vi "MotorInterfaceV2.vi"() -> ()   [LabVIEW 2020]
uses:
  <vilib>/DAQmx/write.llb/DAQmx Write (Digital 1D U16 1Chan NSamp).vi
  <vilib>/DAQmx/create/channels.llb/DAQmx Create Channel (DO-Digital Output).vi
  <vilib>/Waveform/DWDTOps.llb/DWDT Analog to Digital.vi
  <vilib>/Waveform/DWDTOps.llb/DWDT Digital to Binary U16.vi
  <vilib>/DAQmx/configure/timing.llb/DAQmx Timing (Sample Clock).vi
  <vilib>/DAQmx/miscellaneous.llb/DAQmx Fill In Error Info.vi
  <vilib>/measure/NI_MABase.lvlib
panel:
  out "digital waveform":digitalwaveform(waveform)={"t0"=timestamp(0 s since 1904-01-01), "dt"=0.0, "Y"={"transitions"=[], "data"=[]}, "error"={"status"=FALSE, "code"=37421928, "source"=""}}
  out "resolution (out)":i32=16
  out "Waveform Graph":waveform(dbl)(graph)
  in  "frequency":dbl=10.0 format="%0.2p"
  out "Fault":bool
  out "Direction Test\nPort 0_2":bool[](array[boolean])
  out "Reset Test\nPort 0_1":bool[](array[boolean])
  out "Enable Test\nPort 0_0":bool[](array[boolean])
  in  "Direction":bool
  in  "Reset":bool
  in  "Enable":bool
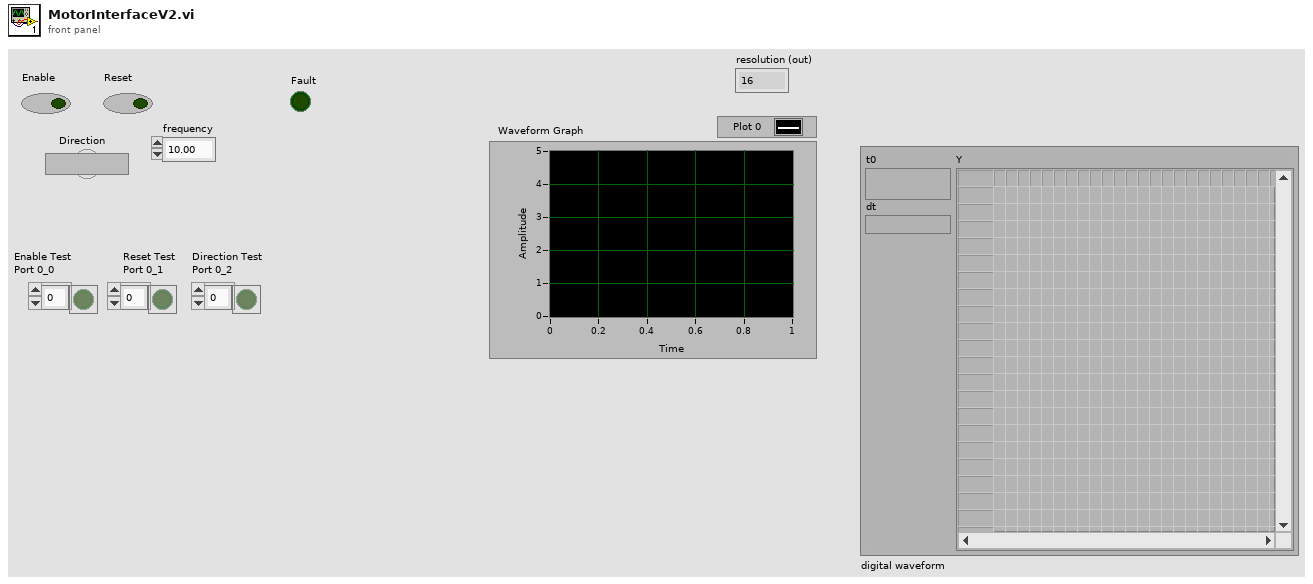
[diagram p1: front panel]
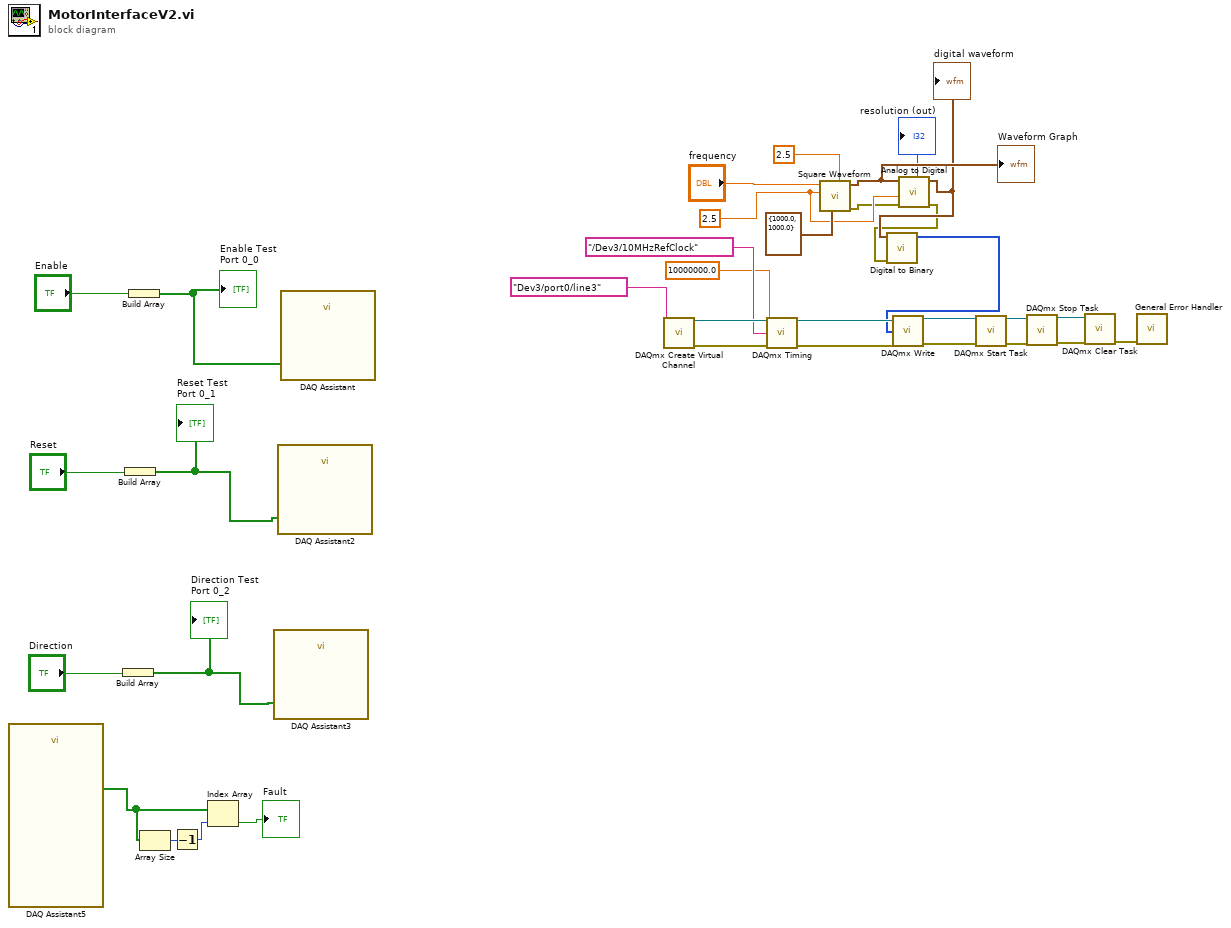
[diagram p0: block diagram]
diagram:
  w14 = 2.5 ("amplitude")
  n1 = call "DAQ Assistant5"() -> ("data"=w27:bool[])  [unwired: 17 in, 2 out]
  n2 = Build Array("Direction") -> (w29:bool[])
  "Direction Test\nPort 0_2" <- w29
  n3 = Build Array("Reset") -> (w31:bool[])
  "Reset Test\nPort 0_1" <- w31
  n4 = Build Array("Enable") -> (w34:bool[])
  "Enable Test\nPort 0_0" <- w34
  n5 = Array Size(array=w27) -> (size(s)=w26:i32)
  n6 = Decrement(x=w26) -> (x-1=w25:i32)
  n7 = Index Array(array=w27, index=w25) -> (element=→"Fault":bool)
  n8 = call "DAQ Assistant3"("data"=w29) -> ()  [unwired: 17 in, 2 out]
  n9 = call "DAQ Assistant2"("data"=w31) -> ()  [unwired: 17 in, 2 out]
  n10 = call "DAQ Assistant"("data"=w34) -> ()  [unwired: 17 in, 2 out]
  n11 = call-poly <vilib>:"DAQmx Create Virtual Channel.vi"("lines"=tag "Dev3/port0/line3") -> ("task out"=w23:refnum<k21>, "error out"=w22:errorcluster)  [unwired: 13 in]
  n12 = call-poly <vilib>:"DAQmx Timing.vi"("task/channels in"=w23, "rate"=10000000.0, "source"=tag "/Dev3/10MHzRefClock", "error in"=w22) -> ("task out"=w10:refnum<k21>, "error out"=w9:errorcluster)  [unwired: 10 in]
  n13 = call <vilib>:"Square Waveform.vi"("offset"=2.5, "sampling info"=cluster{"Fs":dbl, "#s":dbl} {"Fs"=1000.0, "#s"=1000.0}, "amplitude"=w14, "frequency"="frequency") -> ("error out"=w13:errorcluster, "signal out"=w12:waveform(dbl))  [unwired: 6 in]
  "Waveform Graph" <- w12
  n14 = call-poly <vilib>:"Analog to Digital.vi"("error in (no error)"=w13, "full-scale range (pk-pk)"=w14, "analog waveform"=w12) -> ("error out"=w2:errorcluster, "resolution (out)"=→"resolution (out)":i32, "digital waveform"=w3:digitalwaveform)  [unwired: 5 in, 1 out]
  "digital waveform" <- w3
  n15 = call-poly <vilib>:"Digital to Binary.vi"("error in (no error)"=w2, "digital waveform"=w3) -> ("binary array"=w1:u16[])  [unwired: 8 in, 1 out]
  n16 = call-poly <vilib>:"DAQmx Write.vi"("task/channels in"=w10, "data"=w1, "error in"=w9) -> ("task out"=w8:refnum<k21>, "error out"=w7:errorcluster)  [unwired: 10 in, 1 out]
  n17 = call <vilib>:"DAQmx Start Task.vi"("task/channels in"=w8, "error in"=w7) -> ("task out"=w5:refnum<k21>, "error out"=w6:errorcluster)  [unwired: 12 in]
  n18 = call <vilib>:"DAQmx Stop Task.vi"("task/channels in"=w5, "error in"=w6) -> ("task out"=w21:refnum<k21>, "error out"=w20:errorcluster)  [unwired: 12 in]
  n19 = call <vilib>:"DAQmx Clear Task.vi"("task in"=w21, "error in"=w20) -> ("error out"=w19:errorcluster)  [unwired: 13 in]
  n20 = call <vilib>:"General Error Handler.vi"("error in (no error)"=w19) -> ()  [unwired: 10 in, 5 out]
